vi "U2000_USB_PM_Initialize.vi"(8 "error in (no error)":errorcluster, 9 "Reset (True)":bool=TRUE, 10 "ID Query (True)":bool=TRUE, 11 "VISA resource name":refnum<visa-resource-name>) -> (0 "error out":errorcluster, 3 "VISA resource name out":refnum<visa-resource-name>)   [LabVIEW 2014]
doc: "Establishes communication with the instrument and optionally performs an instrument identification query and/or an instrument reset. It also places the instrument in a default state needed for other instrument driver operations. Therefore, call this VI before calling other instrument driver VIs for this instrument. Generally, you need to call the Initialize VI only once at the beginning of an application."
uses:
  <vilib>/regexp/Match Regular Expression.xnode
panel:
  # "(c) 2011-2015 National Instruments.  ALL RIGHTS RESERVED."
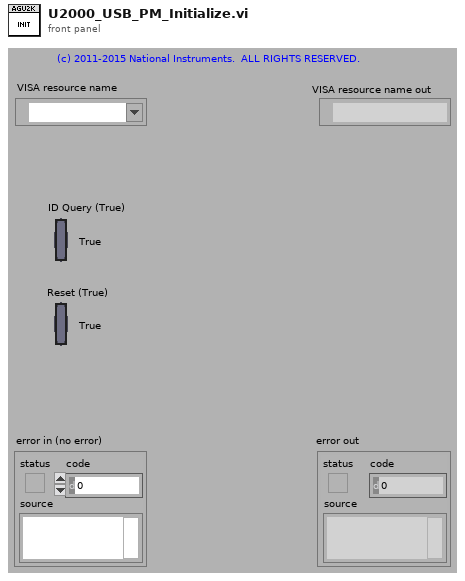
[diagram p1: front panel]
types:
  T1 = cluster{"U2000 Series Mode":u16, "Trigger Source Int/Ext":bool}
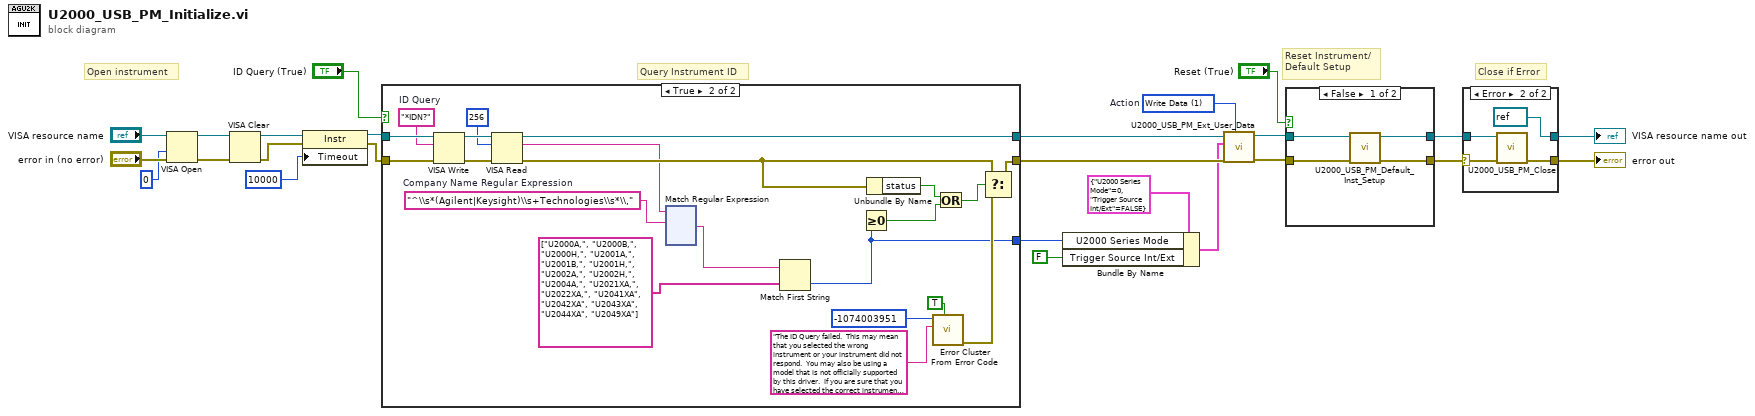
[diagram p0: block diagram]
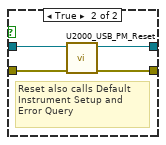
[diagram p3: hidden frame]
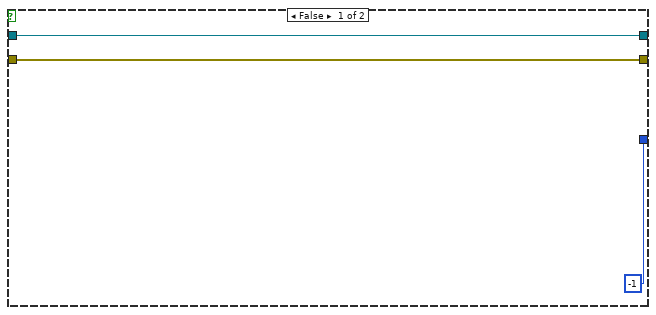
[diagram p4: hidden frame]
diagram:
  w5 = 1 items=["Read Data", "Write Data", "Clear Data", "Clear ALL Data"]  # Action
  # "Close if Error"
  # "Query Instrument ID"
  # "Reset Instrument/\nDefault Setup"
  # "Open instrument"
  n1 = VISA Open(access mode=u32 0, error in (no error)="error in (no error)", VISA resource name="VISA resource name") -> (VISA resource name=w20:refnum<visa-resource-name>, error out=w19:errorcluster)  [unwired: 2 out]
  n2 = VISA Clear(VISA resource name=w20, error in (no error)=w19) -> (VISA resource name out=w14:refnum<visa-resource-name>, error out=w13:errorcluster)
  n3 = property class="Instr"(reference=w14, error in=w13, "Timeout"=u32 10000 ("General Settings:Timeout Value")) -> (reference out=w11:refnum<visa-resource-name>, error out=w10:errorcluster)
  n4 = case shown="True" "ID Query (True)" {
    tunnel: [w27 w49] -> w6
    tunnel: [w28 w46] -> w7
    tunnel: w11 -> [w28 w47]
    tunnel: w10 -> [w27 w48]
    tunnel: [-1 ("index") w32] -> w4
    frame False {
    }
    frame True {
      w29 = "^\\s*(Agilent|Keysight)\\s+Technologies\\s*\\,"  # Company Name Regular Expression
      w42 = "*IDN?"  # ID Query
      n5 = VISA Write(VISA resource name=w47, write buffer=w42, error in (no error)=w48) -> (VISA resource name out=w45:refnum<visa-resource-name>, error out=w44:errorcluster)  [unwired: 1 out]
      n6 = VISA Read(VISA resource name=w45, byte count=u32 256, error in (no error)=w44) -> (VISA resource name out=w46:refnum<visa-resource-name>, read buffer=w31:string, error out=w37:errorcluster)  [unwired: 1 out]
      n7 = xnode "Match Regular Expression"("input string"=w31, "regular expression"=w29) -> ("after match"=w30:string)  [unwired: 4 in, 4 out]
      n8 = Match First String(2:string[] ["U2000A,", "U2000B,", "U2000H,", "U2001A,", "U2001B,", "U2001H,", "U2002A,", "U2002H,", "U2004A,", "U2021XA,", "U2022XA,", "U2041XA", "U2042XA", "U2043XA", "U2044XA", "U2049XA"] ("string array"), 3:w30) -> (0:w32:i32)  [unwired: 1 out]
      n9 = Greater Or Equal To 0?(x=w32) -> (x >= 0?=w35:bool)
      n10 = Unbundle By Name(w37) -> ("status"=w36:bool)
      n11 = call <vilib>:"Error Cluster From Error Code.vi"("show call chain? (False)"=TRUE, "error message (\"\")"="The ID Query failed.  This may mean that you selected the wrong instrument or your instrument did not respond.  You may also be using a model that is not officially supported by this driver.  If you are sure that you have selected the correct instrument and it is responding, try disabling the ID Query." ("Source (VI Name)"), "error code (0)"=-1074003951 ("Code")) -> ("error out"=w41:errorcluster)  [unwired: 1 in, 5 out]
      n12 = Or(x=w36, y=w35) -> (x .or. y?=w34:bool)
      n13 = Select(t=w37, s=w34, f=w41) -> (s? t:f=w49:errorcluster)
    }
  }
  n14 = Bundle By Name(cluster=T1 {"U2000 Series Mode"=0, "Trigger Source Int/Ext"=FALSE} ("output cluster"), "U2000 Series Mode"=w4, "Trigger Source Int/Ext"=FALSE) -> (w2:T1)
  n15 = call "U2000_USB_PM_Ext_User_Data.vi"("Action (1: Write Data)"=w5, "error in (no error)"=w6, "User Data In"=w2, "VISA resource name"=w7) -> ("error out"=w8:errorcluster, "VISA resource name out"=w9:refnum<visa-resource-name>)  [unwired: 5 in, 1 out]
  n16 = case shown="False" "Reset (True)" {
    tunnel: w8 -> [w166 w168]
    tunnel: [w164 w171] -> w15
    tunnel: w9 -> [w167 w169]
    tunnel: [w165 w170] -> w16
    frame False {
      n17 = call "U2000_USB_PM_Default_Inst_Setup.vi"("error in (no error)"=w166, "VISA resource name"=w167) -> ("error out"=w164:errorcluster, "VISA resource name out"=w165:refnum<visa-resource-name>)  [unwired: 8 in]
    }
    frame True {
      # "Reset also calls Default Instrument Setup and Error Query"
      n18 = call "U2000_USB_PM_Reset.vi"("error in (no error)"=w168, "VISA resource name"=w169) -> ("error out"=w171:errorcluster, "VISA resource name out"=w170:refnum<visa-resource-name>)  [unwired: 8 in]
    }
  }
  n19 = case shown="Error" w15 {
    selector: w15 -> [w172 w175]
    tunnel: w16 -> [w173 w176]
    tunnel: [w173 refnum<visa-resource-name> refnum ("VISA resource name out")] -> w18
    tunnel: [w172 w177] -> w17
    frame No Error {
    }
    frame Error {
      n20 = call "U2000_USB_PM_Close.vi"("error in (no error)"=w175, "VISA resource name"=w176) -> ("error out"=w177:errorcluster)  [unwired: 9 in]
    }
  }
  "VISA resource name out" <- w18
  "error out" <- w17
